vi "Connect Loop Async.vi"(11 "TCP Client in":refnum<class "TCP Client.lvclass">) -> ()   [LabVIEW 2020, in "Stream-TCP.lvlib" / "TCP Client.lvclass"]
uses:
  TCP Client.lvclass
  C:/dev/LabVIEW/lv-stream/stream/Endpoint/Endpoint.lvclass
  C:/dev/LabVIEW/lv-stream/stream/Connection/Connection.lvclass
  Connection State.ctl
  lv-stream/stream/Connection State.ctl
  TCP Client.lvclass/TCP Client.ctl
  lv-stream/stream/Endpoint/Endpoint.lvclass
  lv-stream/stream/URI/URI.lvclass
  TCP Stream/TCP Stream.lvclass
  lv-stream/stream/Connection/Connection.lvclass
  lv-stream/stream/Stream.lvlib
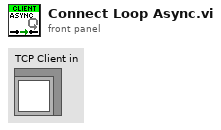
[diagram p1: front panel]
types:
  T1 = typedef "Stream-TCP.lvlib/TCP Client.lvclass/Connection State.ctl" = enum16{"Closed", "Idle", "Connecting", "Connected", "Shutdown"}
  T2 = typedef "Stream.lvlib/Connection State.ctl" = enum16{"Connected", "Disconnected"}
  T3 = typedef "Stream-TCP.lvlib/Client Command.ctl" = enum16{"Connect", "Close", "Shutdown", "Reconnect"}
  T4 = typedef "Stream-TCP.lvlib/Client Command Queue.ctl" = refnum<queue>
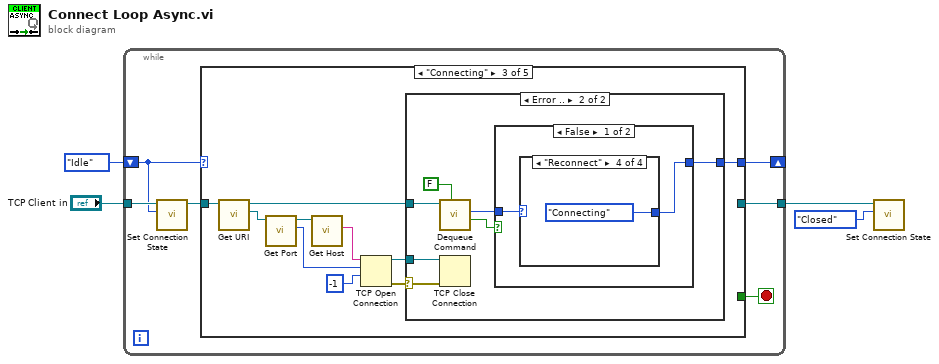
[diagram p0: block diagram]
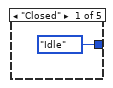
[diagram p2: hidden frame]
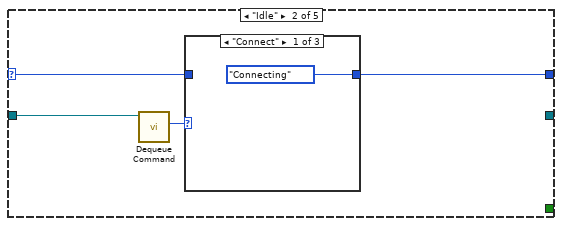
[diagram p3: hidden frame]
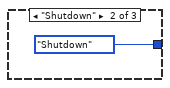
[diagram p4: hidden frame]
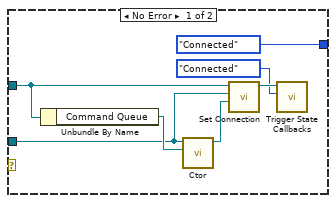
[diagram p6: hidden frame]
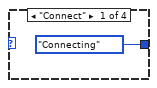
[diagram p7: hidden frame]
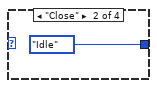
[diagram p8: hidden frame]
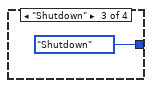
[diagram p9: hidden frame]
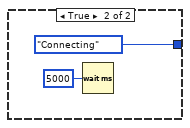
[diagram p10: hidden frame]
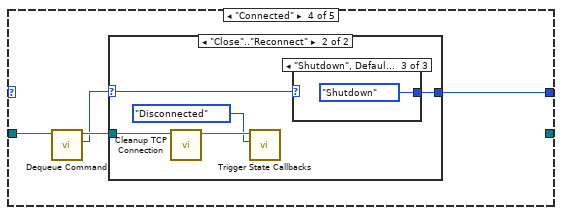
[diagram p11: hidden frame]
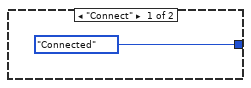
[diagram p12: hidden frame]
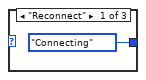
[diagram p13: hidden frame]
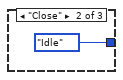
[diagram p14: hidden frame]
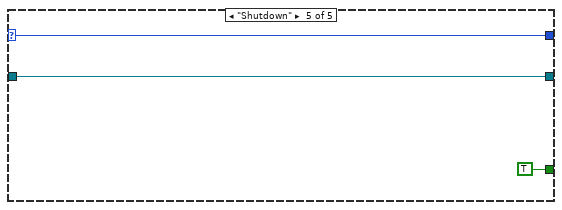
[diagram p15: hidden frame]
diagram:
  n1 = while {
    tunnel: "TCP Client in" -> [w8]
    shift-right: [w5] -> _
    shift-left: Connection_State."Idle" ("Connection State") -> [w6]
    tunnel: [w9] -> w2
    stop <- w10 stop-if-true
    n2 = call "Set Connection State.vi"("Connection State"=w6, "TCP Client in"=w8) -> ("TCP Client out"=w7:refnum<class "TCP Client.lvclass">)  [unwired: 8 in, 1 out]
    n3 = case shown="\"Connecting\"" w6 {
      selector: w6 -> [_ w13 _ _ w64]
      tunnel: [_ _ _ _ TRUE] -> w10
      tunnel: w7 -> [_ w15 w27 w53 w65]
      tunnel: [_ _ _ _ w65] -> w9
      tunnel: [Connection_State."Idle" ("Connection State") w12 w19 w54 w64] -> w5
      frame "Closed" {
      }
      frame "Idle" {
        n4 = call "Dequeue Command.vi"("TCP Client in"=w15) -> ("Command"=w14:T3)  [unwired: 7 in, 3 out]
        n5 = case shown="\"Connect\"" w14 {
          tunnel: [Connection_State."Connecting" ("Connection State") Connection_State."Shutdown" ("Connection State") w18] -> w12
          tunnel: w13 -> [_ _ w18]
          frame "Connect" {
          }
          frame "Shutdown" {
          }
          frame Default {
          }
        }
      }
      frame "Connecting" {
        n6 = call "Get URI.vi"("Endpoint in"=w27) -> ("URI"=w26:refnum<class "URI.lvclass">, "Endpoint out"=w21:refnum<class "TCP Client.lvclass">)  [unwired: 8 in, 1 out]
        n7 = call "Get Port.vi"("URI in"=w26) -> ("Port"=w23:u16, "URI out"=w25:refnum<class "URI.lvclass">)  [unwired: 8 in, 1 out]
        n8 = call "Get Host.vi"("URI in"=w25) -> ("Host"=w24:string)  [unwired: 8 in, 2 out]
        n9 = TCP Open Connection(address=w24, remote port or service name=w23, timeout ms (60000)=-1) -> (connection ID=w20:refnum<k5>, error out=w22:errorcluster)  [unwired: 2 in]
        n10 = case shown="Error .." w22 {
          selector: w22 -> [_ w36]
          tunnel: w21 -> [w33 w41]
          tunnel: w20 -> [w31 w37]
          tunnel: [Connection_State."Connected" ("Connection State") w42] -> w19
          frame No Error {
            n11 = Unbundle By Name(w33) -> ("Command Queue"=w35:T4)
            n12 = call "Ctor.vi"("Client Command Queue"=w35, "TCP Connection"=w31) -> ("TCP Stream out"=w32:refnum<class "TCP Stream.lvclass">)  [unwired: 8 in, 1 out]
            n13 = call "Set Connection.vi"("TCP Stream"=w32, "TCP Connection"=w31, "TCP Client in"=w33) -> ("TCP Client out"=w30:refnum<class "TCP Client.lvclass">)  [unwired: 7 in, 1 out]
            n14 = call "Trigger State Callbacks.vi"("State"=Connection_State."Connected", "Connection in"=w30) -> ()  [unwired: 8 in, 2 out]
          }
          frame Error {
            n15 = call "Dequeue Command.vi"("Wait? (T)"=FALSE, "TCP Client in"=w41) -> ("timed out?"=w39:bool, "Command"=w38:T3)  [unwired: 6 in, 2 out]
            n16 = TCP Close Connection(connection ID=w37, error in (no error)=w36) -> ()  [unwired: 1 in, 2 out]
            n17 = case shown="False" w39 {
              tunnel: [w43 Connection_State."Connecting" ("Connection State")] -> w42
              tunnel: w38 -> [w44 _]
              frame False {
                n18 = case shown="\"Reconnect\"" w44 {
                  tunnel: [Connection_State."Connecting" ("Connection State") Connection_State."Idle" ("Connection State") Connection_State."Shutdown" ("Connection State") Connection_State."Connecting" ("Connection State")] -> w43
                  frame "Connect" {
                  }
                  frame "Close" {
                  }
                  frame "Shutdown" {
                  }
                  frame "Reconnect" {
                  }
                }
              }
              frame True {
                n19 = Wait (ms)(milliseconds to wait=u32 5000) -> ()  [unwired: 1 out]
              }
            }
          }
        }
      }
      frame "Connected" {
        n20 = call "Dequeue Command.vi"("TCP Client in"=w53) -> ("Command"=w51:T3, "TCP Client out"=w52:refnum<class "TCP Client.lvclass">)  [unwired: 7 in, 2 out]
        n21 = case shown="\"Close\"..\"Reconnect\"" w51 {
          selector: w51 -> [_ w56]
          tunnel: [Connection_State."Connected" ("Connection State") w60] -> w54
          tunnel: w52 -> [_ w57]
          frame "Connect" {
          }
          frame "Close".."Reconnect" {
            n22 = call "Cleanup TCP Connection.vi"("TCP Client in"=w57) -> ("TCP Client out"=w59:refnum<class "TCP Client.lvclass">)  [unwired: 9 in, 1 out]
            n23 = call "Trigger State Callbacks.vi"("State"=Connection_State."Disconnected", "Connection in"=w59) -> ()  [unwired: 8 in, 2 out]
            n24 = case shown="\"Shutdown\", Default" w56 {
              tunnel: [Connection_State."Connecting" ("Connection State") Connection_State."Idle" ("Connection State") Connection_State."Shutdown" ("Connection State")] -> w60
              frame "Reconnect" {
              }
              frame "Close" {
              }
              frame "Shutdown", Default {
              }
            }
          }
        }
      }
      frame "Shutdown" {
      }
    }
  }
  n25 = call "Set Connection State.vi"("Connection State"=Connection_State."Closed", "TCP Client in"=w2) -> ()  [unwired: 8 in, 2 out]
